vi "PlotGrid.vi"(6 "Size (um)":u32[](array[numeric]), 9 "No Neurons":i32, 11 "Grid in":refnum<class "Grid.lvclass">) -> (3 "Scene Object Out":refnum<vi>)   [LabVIEW 2013]
uses:
  Cube/Grid.lvclass
  Cube/Grid.lvclass/Grid.ctl
  Neuron/Neuron.lvclass/Neuron.ctl
  Neuron/Get Neuron Properties.vi
  <vilib>/picture/3D Picture Control/Object/Create Object (name).vi
  <vilib>/picture/3D Picture Control/Object/Add Object (no reference).vi
  id2coor.vi
  <vilib>/picture/3D Picture Control/NI_3D Picture Control.lvlib
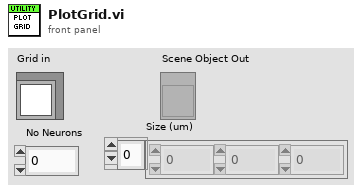
[diagram p1: front panel]
types:
  T1 = enum16{"Normal Bin", "Opaque Bin", "Transparent Bin"}
  T2 = cluster{"Red":sgl, "Green":sgl, "Blue":sgl, "Alpha":sgl}
  T3 = cluster{"[0]":sgl, "[1]":sgl, "[2]":sgl, "[3]":sgl}
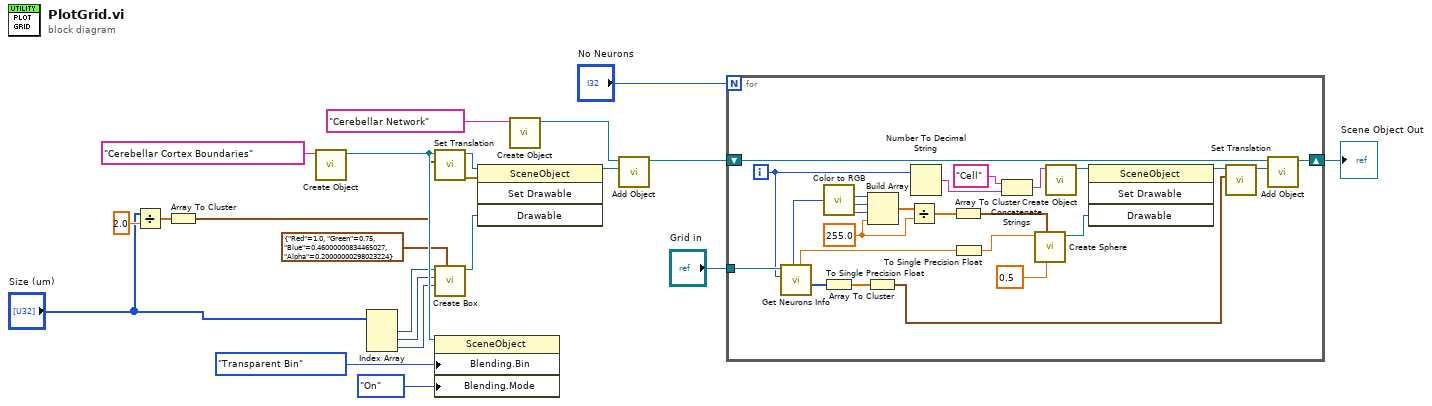
[diagram p0: block diagram]
diagram:
  n1 = Divide(x="Size (um)", y=2.0 ("Numeric")) -> (x/y=w3:dbl[])
  n2 = Array To Cluster(array=w3) -> (cluster=w1:cluster{"[0]":dbl, "[1]":dbl, "[2]":dbl})
  n3 = call-poly <vilib>:"Create Object.vi"("Name"="Cerebellar Cortex Boundaries") -> ("Scene:New Object"=w19:refnum<vi>)  [unwired: 9 in, 1 out]
  n4 = Index Array(array="Size (um)") -> (element #1=w7:u32, element #2=w8:u32, element #3=w9:u32)  [unwired: 3 in]
  n5 = call <vilib>:"Set Translation.vi"("Translation"=w1, "Scene Object"=w19) -> ("error out"=w17:errorcluster, "Translated Object"=w15:refnum<vi>)  [unwired: 8 in]
  n6 = call <vilib>:"Create Box.vi"("Color"=T2 {"Red"=1.0, "Green"=0.75, "Blue"=0.46, "Alpha"=0.2}, "Length Z"=w9, "Length Y"=w8, "Length X"=w7) -> ("New Box Refnum"=w5:refnum<vi>)  [unwired: 6 in, 1 out]
  n7 = property class="SceneObject"(reference=w19, "Blending.Bin"=T1."Transparent Bin" ("Blending:Bin"), "Blending.Mode"=enum16{"Inherit Value", "Off", "On"}."On" ("Blending:Mode")) -> ()  [unwired: 1 in, 2 out]
  n8 = invoke class="SceneObject" method="Set Drawable"(reference=w15, error in=w17, "Drawable"=w5) -> (reference out=w12:refnum<vi>)  [unwired: 1 in, 3 out]
  n9 = call-poly <vilib>:"Create Object.vi"("Name"="Cerebellar Network") -> ("Scene:New Object"=w11:refnum<vi>)  [unwired: 9 in, 1 out]
  n10 = call-poly <vilib>:"Add Object.vi"("New Object In"=w12, "Scene Object In"=w11) -> ("Scene Object Out"=w10:refnum<vi>)  [unwired: 8 in, 1 out]
  n11 = for {
    N: "No Neurons" -> [_]
    shift-right: [w45] -> w20
    shift-left: w10 -> [w44]
    tunnel: "Grid in" -> [w40]
    i -> [w35]
    w27 = sgl 255.0 ("Detail")
    n12 = call "Get Neurons Info.vi"("Neuron No"=w35, "Grid in"=w40) -> ("Position"=w39:i32[], "Size radio (um)"=w33:dbl, "Color"=w32:u32)  [unwired: 3 in, 4 out]
    n13 = call <vilib>:"Color to RGB.vi"("Color"=w32) -> ("R"=w31:u8, "G"=w30:u8, "B"=w29:u8)  [unwired: 1 out]
    n14 = To Single Precision Float(number=w39) -> (single precision float=w24:sgl[])
    n15 = Array To Cluster(array=w24) -> (cluster=w23:cluster{"[0]":sgl, "[1]":sgl, "[2]":sgl})
    n16 = Build Array(w31, w30, w29, w27) -> (w28:sgl[])
    n17 = Divide(x=w28, y=w27) -> (x/y=w26:sgl[])
    n18 = Number To Decimal String(number=w35) -> (decimal integer string=w36:string)  [unwired: 1 in]
    n19 = Array To Cluster(array=w26) -> (cluster=w25:T3)
    n20 = To Single Precision Float(number=w33) -> (single precision float=w34:sgl)
    n21 = Concatenate Strings("Cell" ("Name"), w36) -> (w38:string)
    n22 = call <vilib>:"Create Sphere.vi"("Detail"=sgl 0.5, "Color"=w25, "Radius"=w34) -> ("New Sphere Refnum"=w46:refnum<vi>)  [unwired: 7 in, 1 out]
    n23 = call-poly <vilib>:"Create Object.vi"("Name"=w38) -> ("Scene:New Object"=w47:refnum<vi>)  [unwired: 9 in, 1 out]
    n24 = invoke class="SceneObject" method="Set Drawable"(reference=w47, "Drawable"=w46) -> (reference out=w43:refnum<vi>)  [unwired: 2 in, 3 out]
    n25 = call <vilib>:"Set Translation.vi"("Translation"=w23, "Scene Object"=w43) -> ("Translated Object"=w42:refnum<vi>)  [unwired: 8 in, 1 out]
    n26 = call-poly <vilib>:"Add Object.vi"("New Object In"=w42, "Scene Object In"=w44) -> ("Scene Object Out"=w45:refnum<vi>)  [unwired: 8 in, 1 out]
  }
  "Scene Object Out" <- w20
